vi "puertosIP.vi"(8 "error in (no error)":errorcluster) -> (0 "error out":errorcluster, 1 "Cluster":T1={"IMonWeb"="http://195.77.159.50:8008/IMon.txt", "IMon"=TRUE, "VMonWeb"="http://195.77.159.50:8008/VMon.txt", "VMon"=TRUE, "ClimatWeb"="http://195.77.159.50:8008/clim.txt", "Climat"=TRUE, "RadonWeb"="http://localhost:90/radon.txt", "Radon"=TRUE, "BeagleEWeb"="http://192.168.3.90:8080/anaisElect.txt", "BeagleE"=TRUE, "BeagleDWeb"="http://192.168.3.91:8080/anaisDet.txt", "BeagleD"=TRUE, "RateWeb"="http://195.77.159.50:8008/rate.txt", "Rate"=TRUE, "CratesWeb"="http://195.77.159.50:8008/crates.txt", "Crates"=TRUE, "StartStopWeb"="", "StartStop"=TRUE, "MuonRatesWeb"="", "MuonRates"=TRUE, "N2LIQWeb"="", "N2LIQ"=TRUE}, 2 "VISA radon 2":refnum<visa-resource-name>="COM35")   [LabVIEW 2013]
uses:
  puertosIP.ctl
panel:
  in  "VISA radon":refnum<visa-resource-name>="COM35"
  in  "ClusterIN":T1={"IMonWeb"="http://195.77.159.50:8008/IMon.txt", "IMon"=TRUE, "VMonWeb"="http://195.77.159.50:8008/VMon.txt", "VMon"=TRUE, "ClimatWeb"="http://195.77.159.50:8008/clim.txt", "Climat"=TRUE, "RadonWeb"="http://localhost/radon.txt", "Radon"=TRUE, "BeagleEWeb"="http://192.168.3.90:8080/anaisElect.txt", "BeagleE"=TRUE, "BeagleDWeb"="http://192.168.3.91:8080/anaisDet.txt", "BeagleD"=TRUE, "RateWeb"="http://195.77.159.50:8008/rate.txt", "Rate"=TRUE, "CratesWeb"="http://195.77.159.50:8008/crates.txt", "Crates"=TRUE, "StartStopWeb"="http://195.77.159.50:8008/startstop.txt", "StartStop"=TRUE, "MuonRatesWeb"="http://195.77.159.50:8008/muonrateSidescontrol.txt", "MuonRates"=TRUE, "N2LIQWeb"="http://localhost/N2Control.txt", "N2LIQ"=TRUE}
  out "Si usado":bool=TRUE
  out "No usado":bool
  in  "stop":bool
  # "http://193.146.122.114:80/radon.txt"
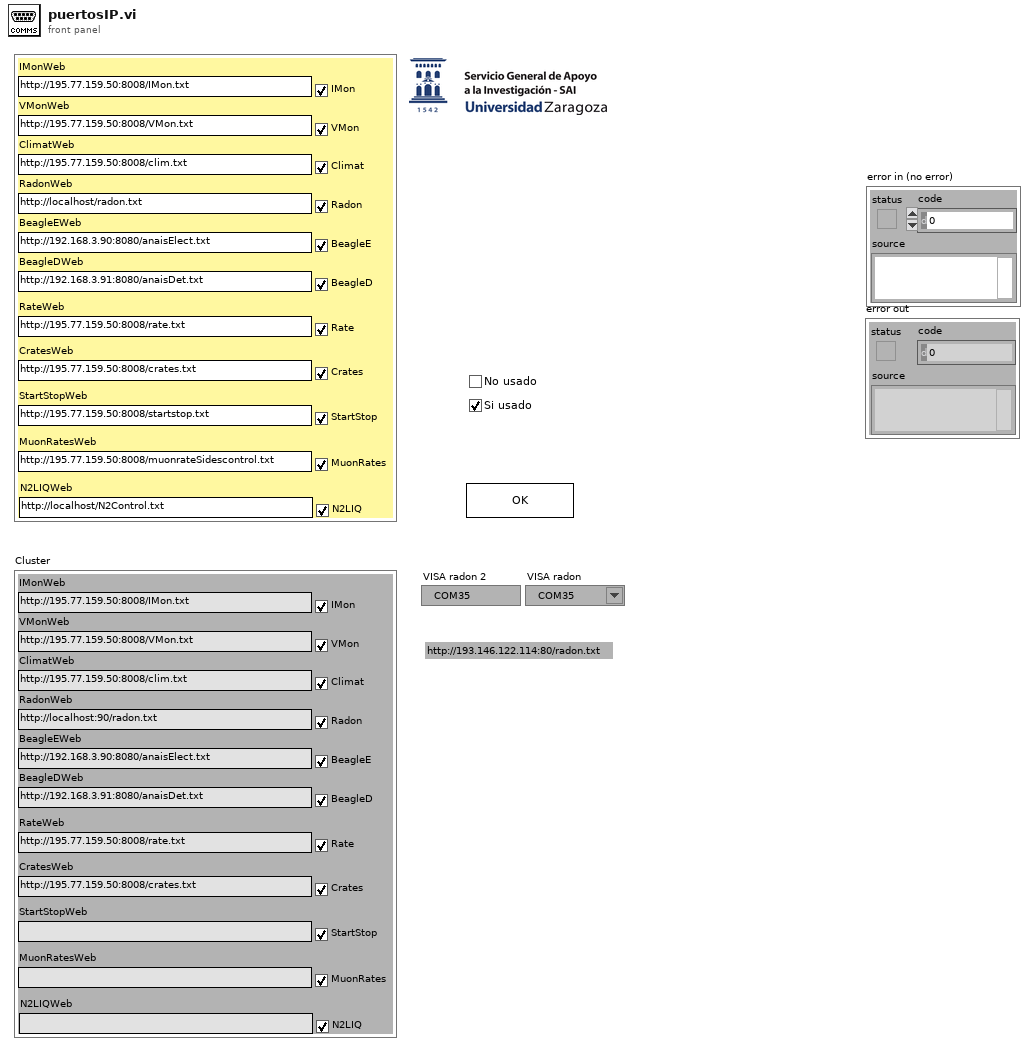
[diagram p1: front panel]
types:
  T1 = typedef "puertosIP.ctl" = cluster{"IMonWeb":string, "IMon":bool, "VMonWeb":string, "VMon":bool, "ClimatWeb":string, "Climat":bool, "RadonWeb":string, "Radon":bool, "BeagleEWeb":string, "BeagleE":bool, "BeagleDWeb":string, "BeagleD":bool, "RateWeb":string, "Rate":bool, "CratesWeb":string, "Crates":bool, "StartStopWeb":string, "StartStop":bool, "MuonRatesWeb":string, "MuonRates":bool, "N2LIQWeb":string, "N2LIQ":bool}
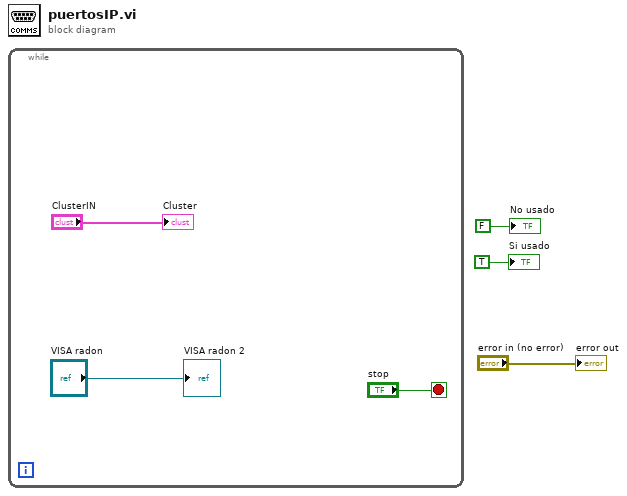
[diagram p0: block diagram]
diagram:
  n1 = while {
    stop <- "stop" stop-if-true
    "Cluster" <- "ClusterIN"
    "VISA radon 2" <- "VISA radon"
  }
  "No usado" <- FALSE ("No usado")
  "Si usado" <- TRUE ("Si usado")
  "error out" <- "error in (no error)"
